vi "radar.vi"() -> ()   [LabVIEW 2020]
uses:
  88a7b435-938b-43aa-a90b-41551c91a520.vi
  9e44051b-2116-4b69-b735-51434e18ac48.vi
  <vilib>/Instr/_visa.llb/VISA Configure Serial Port (Instr).vi
panel:
  out "Meter":dbl(knob) scale=0.0..100.0
  out "length":i32
  out "Waveform Chart":cluster{"type":u16, i32}(graph)
  out "XY Graph":cluster{sgl[], sgl[]}(graph)
  out "n_of_point_data":u16(slide) scale=0.0..100.0
  out "n_of_frame":u32
  out "header_2":u16 format="%.0x"
  out "header_1":u16 format="%.0x"
  out "packet_size":u32(slide) scale=0.0..1000.0
  out "Numeric":i32
  in  "stop":bool
  out "concatenated string":string
  out "error out":errorcluster
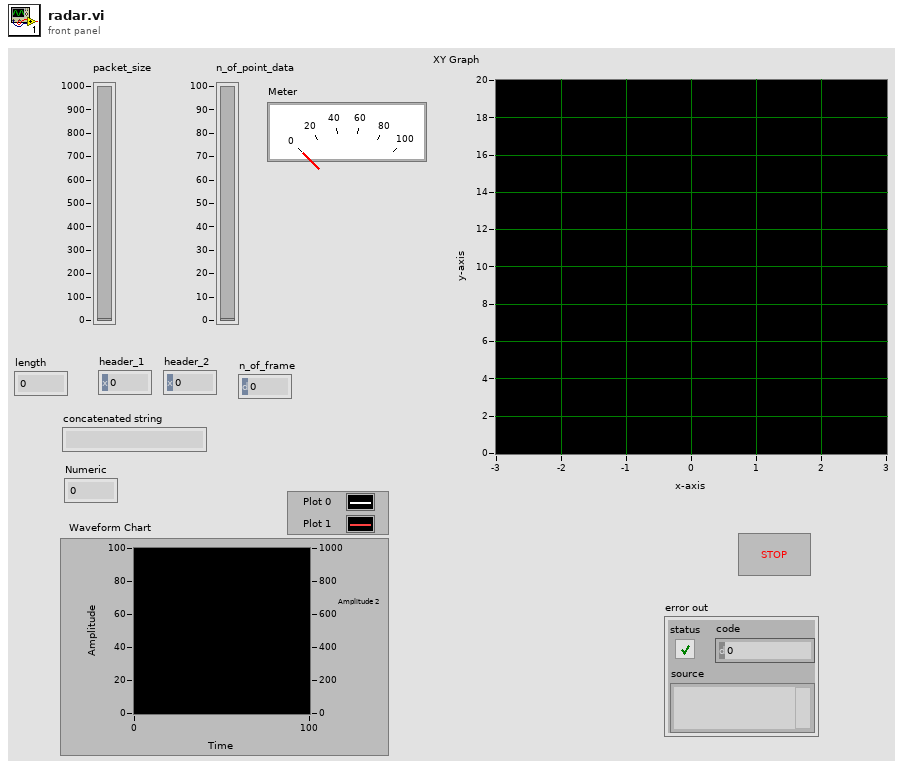
[diagram p1: front panel]
types:
  T1 = enum16{"big-endian, network order", "native, host order", "little-endian"}
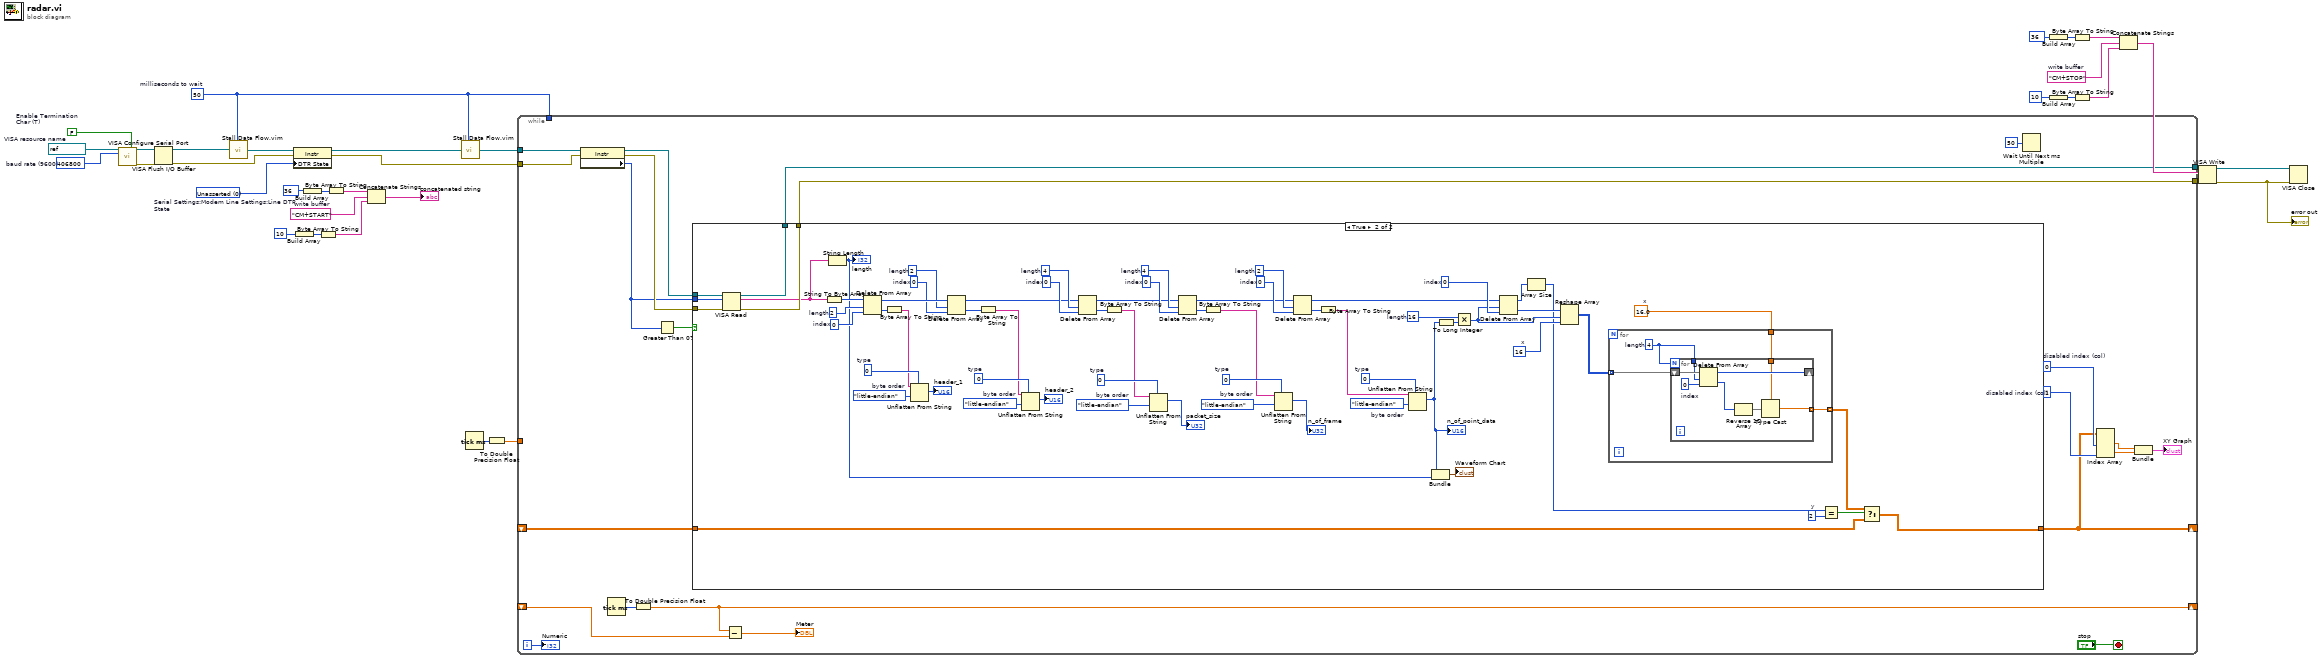
[diagram p0: block diagram]
diagram:
  w17 = "CM+STOP"  # write buffer
  w21 = i16 0 items=["Unknown"=-1, "Unasserted"=0, "Asserted"=1]  # Serial Settings:Modem Line Settings:Line DTR State
  w27 = FALSE  # Enable Termination Char (T)
  w5 = u32 50  # milliseconds to wait
  w28 = "CM+START"  # write buffer
  w34 = u32 406800  # baud rate (9600)
  w35 = refnum<visa-resource-name> "COM3"  # VISA resource name
  n1 = call-poly "VISA Configure Serial Port"("VISA resource name"=w35, "Enable Termination\nChar (T)"=w27, "baud rate (9600)"=w34) -> ("VISA resource name out"=w33:refnum<visa-resource-name>, "error out"=w32:errorcluster)  [unwired: 11 in]
  n2 = VISA Flush I/O Buffer(VISA resource name=w33, error in (no error)=w32) -> (VISA resource name out=w8:refnum<visa-resource-name>, error out=w6:errorcluster)  [unwired: 1 in]
  n3 = call "Stall Data Flow.vim"("value in"=w8, "milliseconds to wait"=w5) -> ("value out"=w7:refnum<visa-resource-name>)  [unwired: 1 out]
  n4 = property class="Instr"(reference=w7, error in=w6, "DTR State"=w21) -> (reference out=w4:refnum<visa-resource-name>, error out=w3:errorcluster)
  n5 = Build Array(u8 10) -> (w24:u8[])
  n6 = Build Array(u8 36) -> (w30:u8[])
  n7 = Byte Array To String(unsigned byte array=w24) -> (string=w22:string)
  n8 = Byte Array To String(unsigned byte array=w30) -> (string=w29:string)
  n9 = Concatenate Strings(w29, w28, w22) -> (→"concatenated string":string)
  n10 = call "Stall Data Flow.vim"("value in"=w4, "milliseconds to wait"=w5) -> ("value out"=w25:refnum<visa-resource-name>)  [unwired: 1 out]
  n11 = Tick Count (ms)() -> (millisecond timer value=w2:u32)
  n12 = To Double Precision Float(number=w2) -> (double precision float=w1:dbl)
  n13 = while {
    tunnel: [w50] -> w11
    tunnel: [w51] -> w12
    tunnel: w3 -> [w48]
    tunnel: w25 -> [w43]
    shift-right: [w36] -> _
    shift-left: _ -> [w49]
    tunnel: w5 -> [_]
    shift-right: [w44] -> _
    shift-left: _ -> [w46]
    tunnel: w1 -> [_]
    i -> [w56]
    stop <- "stop" stop-if-true
    w37 = 1  # disabled index (col)
    w38 = 0  # disabled index (col)
    n14 = property class="Instr"(reference=w43, error in=w48) -> (reference out=w54:refnum<visa-resource-name>, error out=w53:errorcluster, "Serial Settings:Number of Bytes at Serial Port"=w52:u32)
    n15 = Tick Count (ms)() -> (millisecond timer value=w47:u32)
    n16 = To Double Precision Float(number=w47) -> (double precision float=w44:dbl)
    n17 = Greater Than 0?(x=w52) -> (x > 0?=w55:bool)
    n18 = case shown="True" w55 {
      tunnel: w54 -> [w60 w76]
      tunnel: w53 -> [w59 w75]
      tunnel: w52 -> [_ w74]
      tunnel: [w60 w73] -> w51
      tunnel: [w59 w72] -> w50
      tunnel: [w58 w67] -> w36
      tunnel: w49 -> [w58 w66]
      frame False {
      }
      frame True {
        w65 = sgl 16.0  # x
        w70 = 2  # y
        w79 = 16  # x
        w84 = 0  # index
        w85 = 16  # length
        w87 = u16 0  # type
        w88 = T1."little-endian"  # byte order
        w91 = 0  # index
        w90 = 2  # length
        w96 = u32 0  # type
        w95 = T1."little-endian"  # byte order
        w98 = 0  # index
        w99 = 4  # length
        w104 = u32 0  # type
        w105 = T1."little-endian"  # byte order
        w108 = 0  # index
        w107 = 4  # length
        w113 = u16 0  # type
        w112 = T1."little-endian"  # byte order
        w115 = 0  # index
        w116 = 2  # length
        w119 = 0  # index
        w120 = 2  # length
        w123 = u16 0  # type
        w124 = T1."little-endian"  # byte order
        n19 = VISA Read(VISA resource name=w76, byte count=w74, error in (no error)=w75) -> (VISA resource name out=w73:refnum<visa-resource-name>, read buffer=w61:string, error out=w72:errorcluster)  [unwired: 1 out]
        n20 = String To Byte Array(string=w61) -> (unsigned byte array=w121:u8[])
        n21 = String Length(string=w61) -> (length=w62:i32)
        "length" <- w62
        n22 = Delete From Array(array=w121, length=w120, index=w119) -> (deleted portion=w118:u8[], array with subset deleted=w117:u8[])
        n23 = Byte Array To String(unsigned byte array=w118) -> (string=w111:string)
        n24 = Unflatten From String(type=w123, binary string=w111, byte order (0:big-endian, network order)=w124) -> (value=→"header_1":u16)  [unwired: 2 in, 2 out]
        n25 = Delete From Array(array=w117, length=w116, index=w115) -> (deleted portion=w110:u8[], array with subset deleted=w106:u8[])
        n26 = Byte Array To String(unsigned byte array=w110) -> (string=w109:string)
        n27 = Unflatten From String(type=w113, binary string=w109, byte order (0:big-endian, network order)=w112) -> (value=→"header_2":u16)  [unwired: 2 in, 2 out]
        n28 = Delete From Array(array=w106, length=w107, index=w108) -> (deleted portion=w103:u8[], array with subset deleted=w97:u8[])
        n29 = Byte Array To String(unsigned byte array=w103) -> (string=w102:string)
        n30 = Unflatten From String(type=w104, binary string=w102, byte order (0:big-endian, network order)=w105) -> (value=→"packet_size":u32)  [unwired: 2 in, 2 out]
        n31 = Delete From Array(array=w97, length=w99, index=w98) -> (deleted portion=w100:u8[], array with subset deleted=w89:u8[])
        n32 = Byte Array To String(unsigned byte array=w100) -> (string=w94:string)
        n33 = Unflatten From String(type=w96, binary string=w94, byte order (0:big-endian, network order)=w95) -> (value=→"n_of_frame":u32)  [unwired: 2 in, 2 out]
        n34 = Delete From Array(array=w89, length=w90, index=w91) -> (deleted portion=w92:u8[], array with subset deleted=w83:u8[])
        n35 = Byte Array To String(unsigned byte array=w92) -> (string=w86:string)
        n36 = Unflatten From String(type=w87, binary string=w86, byte order (0:big-endian, network order)=w88) -> (value=w64:u16)  [unwired: 2 in, 2 out]
        "n_of_point_data" <- w64
        n37 = Bundle("type"=w64, w62) -> (→"Waveform Chart":cluster{"type":u16, i32})  [unwired: 1 in]
        n38 = To Long Integer(number=w64) -> (32bit integer=w82:i32)
        n39 = Multiply(x=w85, y=w82) -> (x*y=w78:i32)
        n40 = Delete From Array(array=w83, length=w78, index=w84) -> (deleted portion=w80:u8[], array with subset deleted=w81:u8[])
        n41 = Array Size(array=w81) -> (size(s)=w71:i32)
        n42 = Reshape Array "Reshape Array"(w80, w78, w79) -> (w77:u8[][])
        n43 = for {
          tunnel: w77 -> [w128] mode=indexing
          tunnel: [w126] -> w68 mode=indexing
          tunnel: w65 -> [w125]
          w127 = 4  # length
          n44 = for {
            N: w127 -> [_]
            tunnel: w127 -> [w135]
            shift-right: [w133] -> _
            shift-left: w128 -> [w136]
            tunnel: [w132] -> w126 mode=indexing
            tunnel: w125 -> [w129]
            w134 = 0  # index
            n45 = Delete From Array(array=w136, length=w135, index=w134) -> (deleted portion=w131:u8[], array with subset deleted=w133:u8[])
            n46 = Reverse 1D Array(array=w131) -> (reversed array=w130:u8[])
            n47 = Type Cast(type=w129, x=w130) -> (*(type *) &x=w132:sgl)
          }
        }
        n48 = Equal?(x=w71, y=w70) -> (x = y?=w69:bool)
        n49 = Select(t=w68, s=w69, f=w66) -> (s? t:f=w67:sgl[][])
      }
    }
    n50 = Subtract(x=w44, y=w46) -> (x-y=→"Meter":dbl)
    n51 = Wait Until Next ms Multiple(millisecond multiple=u32 50) -> ()  [unwired: 1 out]
    n52 = Index Array(array=w36, index (col) #1=w38, index (col) #2=w37) -> (element #1=w39:sgl[], element #2=w41:sgl[])  [unwired: 2 in]
    n53 = Bundle(w39, w41) -> (→"XY Graph":cluster{sgl[], sgl[]})  [unwired: 1 in]
    "Numeric" <- w56
  }
  n54 = Build Array(u8 36) -> (w15:u8[])
  n55 = Build Array(u8 10) -> (w18:u8[])
  n56 = Byte Array To String(unsigned byte array=w15) -> (string=w16:string)
  n57 = Byte Array To String(unsigned byte array=w18) -> (string=w20:string)
  n58 = Concatenate Strings(w16, w17, w20) -> (w13:string)
  n59 = VISA Write(VISA resource name=w12, write buffer=w13, error in (no error)=w11) -> (VISA resource name out=w10:refnum<visa-resource-name>, error out=w9:errorcluster)  [unwired: 1 out]
  "error out" <- w9
  n60 = VISA Close(VISA resource name=w10, error in (no error)=w9) -> ()  [unwired: 1 out]
